vi "CAN ISA Close.vi"() -> (0 "Error Number":u32 format="%.0x")   [LabVIEW 2009]
doc: "Schliest die Verbindung zur Hardware."
uses:
  PCAN_ISA.dll
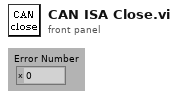
[diagram p1: front panel]
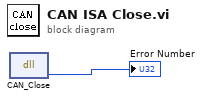
[diagram p0: block diagram]
diagram:
  n1 = dll-call lib="C:/Documents and Settings/PQ/Desktop/LabView-Dateien/PCAN_ISA.dll" fn="CAN_Close" label="CAN_Close (void)"() -> ("Error Number"=→"Error Number":u32)  [unwired: 3 in, 2 out]
